vi "Register Backlog.vi"(7 "TimingEngine":T2, 8 "error in (no error)":errorcluster, 9 "DAQ Diag":T1, 10 "Task Name":string, 11 "FP Controls in":refnum<class "FP Controls.lvclass">) -> (0 "error out":errorcluster, 3 "FP Controls out":refnum<class "FP Controls.lvclass">)   [LabVIEW 2018, in "Configuration Grandmaster.lvlib" / "FP Controls.lvclass"]
uses:
  FP Controls.lvclass
  Common/Controls/TE_Designator.ctl
  Common/Controls/DAQ Diagnostics.ctl
  FP Controls.lvclass/FP Controls.ctl
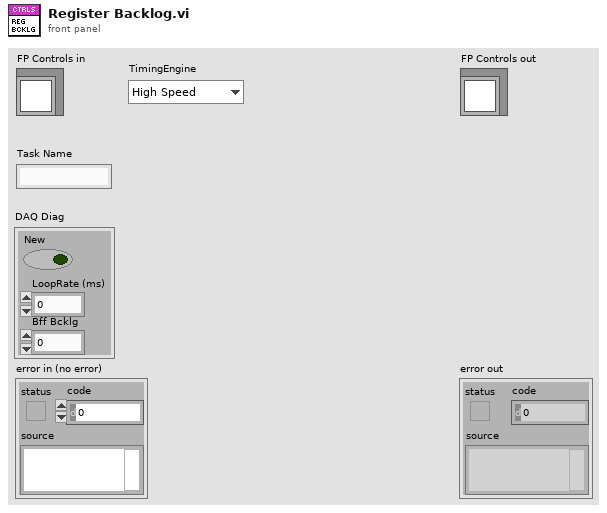
[diagram p1: front panel]
types:
  T1 = typedef "DAQ Diagnostics.ctl" = cluster{"New":bool, "LoopRate (ms)":u32, "Bff Bcklg":dbl}
  T2 = typedef "TE_Designator.ctl" = enum16{"High Speed", "Low Speed"}
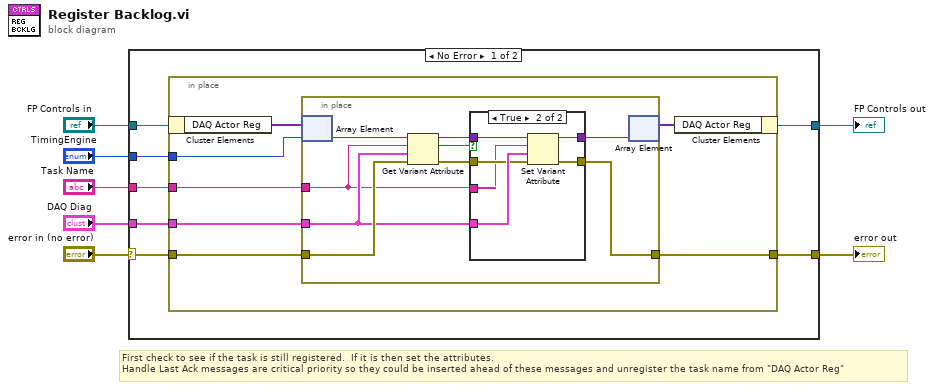
[diagram p0: block diagram]
diagram:
  # "First check to see if the task is still registered.  If it is then set the attributes.\nHandle Last Ack messages are critical priority so they could be inserted ahead of these messages and unregister the task name from \"DAQ Actor Reg\""
  n1 = case shown="No Error" "error in (no error)" {
    selector: "error in (no error)" -> [w14 w40]
    tunnel: [w13 w40] -> w6
    tunnel: [w8 w39] -> w4
    tunnel: "FP Controls in" -> [w10 w39]
    tunnel: "DAQ Diag" -> [w12 _]
    tunnel: "Task Name" -> [w11 _]
    tunnel: "TimingEngine" -> [w9 _]
    frame No Error {
      n2 = in-place {
        in-place-border: w14 -> [w21]
        in-place-border: [w20] -> w13
        in-place-border: w12 -> [w19]
        in-place-border: w11 -> [w18]
        in-place-border: w9 -> [w16]
        n3 = in-place-cluster #1(w10) -> ("DAQ Actor Reg"=w17:variant[])
        n4 = in-place {
          in-place-border: w21 -> [w27]
          in-place-border: [w24] -> w20
          in-place-border: w19 -> [w26]
          in-place-border: w18 -> [w22]
          n5 = in-place-array #2(w17, w16) -> (w29:variant)
          n6 = Get Variant Attribute(Variant=w29, name=w22, default value (empty Variant)=w26, error in=w27) -> (duplicate Variant=w28:variant, found=w23:bool, error out=w25:errorcluster)  [unwired: 1 out]
          n7 = case shown="True" w23 {
            tunnel: [w32 w38] -> w30
            tunnel: w28 -> [w32 w37]
            tunnel: w26 -> [_ w36]
            tunnel: w25 -> [w31 w35]
            tunnel: [w31 w34] -> w24
            tunnel: w22 -> [_ w33]
            frame False {
            }
            frame True {
              n8 = Set Variant Attribute(Variant=w37, name=w33, value=w36, error in=w35) -> (Variant out=w38:variant, error out=w34:errorcluster)  [unwired: 1 out]
            }
          }
          n9 = in-place-array #2(w30) -> (w15:variant[])  [unwired: 1 out]
        }
        n10 = in-place-cluster #1("DAQ Actor Reg"=w15) -> (w8:refnum<class "FP Controls.lvclass">)
      }
    }
    frame Error {
    }
  }
  "error out" <- w6
  "FP Controls out" <- w4
